vi "ReadRestart.vi"(8 "error in (no error)":errorcluster, 11 "object in":refnum<class "shutdown_request Message.lvclass">) -> (0 "error out":errorcluster, 2 "restart":bool, 3 "object out":refnum<class "shutdown_request Message.lvclass">)   [LabVIEW 2018, in "ClientMessaging.lvlib" / "shutdown_request Message.lvclass"]
uses:
  shutdown_request Message.lvclass
  shutdown_request Message.lvclass/shutdown_request Message.ctl
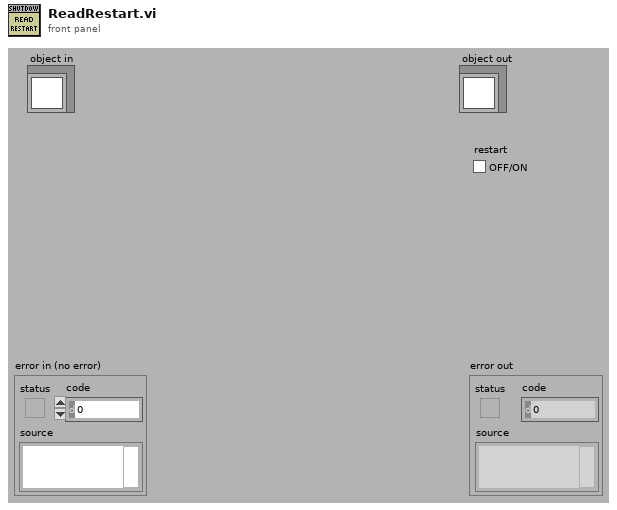
[diagram p1: front panel]
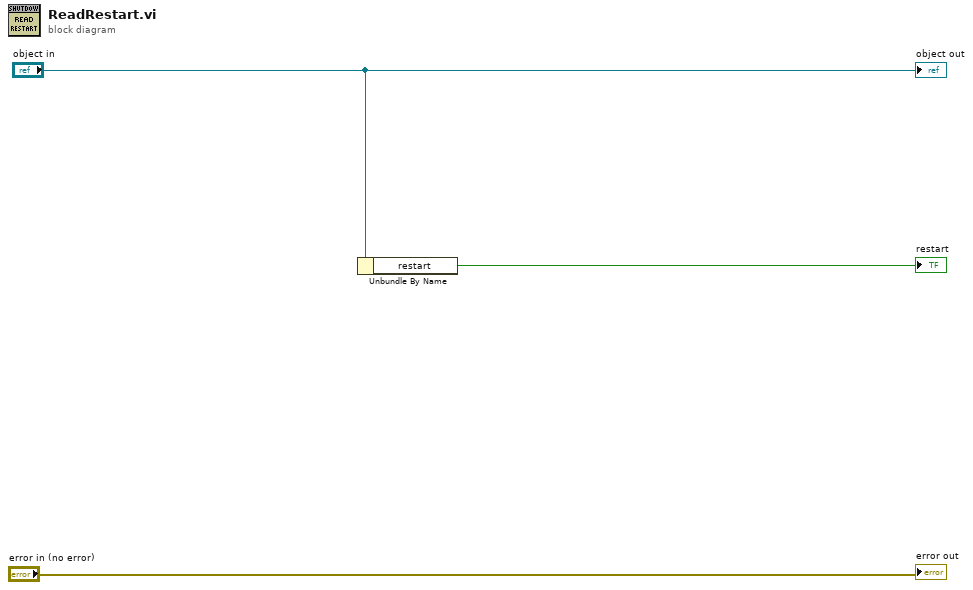
[diagram p0: block diagram]
diagram:
  n1 = Unbundle By Name("object in") -> ("restart"=→"restart":bool)
  "error out" <- "error in (no error)"
  "object out" <- "object in"
